vi "xijk_check_path_is_empty.vi"(10 "Excitation filter 2":path, 11 "Path":path) -> (2 "Excitation filter 1":path)   [LabVIEW 2010]
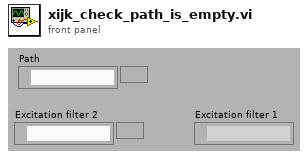
[diagram p1: front panel]
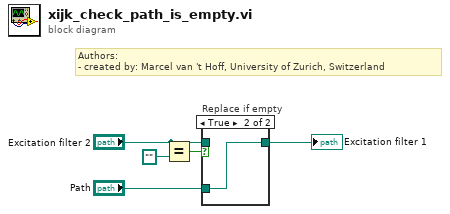
[diagram p0: block diagram]
diagram:
  # "Authors: \n- created by: Marcel van 't Hoff, University of Zurich, Switzerland"
  n1 = Equal?(x="Excitation filter 2", y=path "") -> (x = y?=w4:bool)
  n2 = case "Replace if empty" shown="True" w4 {
    tunnel: "Path" -> [_ w7]
    tunnel: "Excitation filter 2" -> [w6 _]
    tunnel: [w6 w7] -> w5
    frame False {
    }
    frame True {
    }
  }
  "Excitation filter 1" <- w5
